vi "peak detector logic tester.vi"() -> ()   [LabVIEW 2021]
uses:
  <vilib>/rvi/FXPMathLib/FxpRectToPolar/subVIs/nifxpmath_RectToPolar_SimConfig.ctl
  <vilib>/rvi/Emulation/niFpgaSctlEmulationGetInTimedLoop.vi
  <vilib>/rvi/FXPMathLib/FxpRectToPolar/simVIs/DllFxpRectToPolarTemp_sub.vi
  <vilib>/rvi/Memory/Memory_Emulation/nirvimemoryFastEmulation.vi
  <vilib>/rvi/Memory/Memory_Emulation/nirvimemoryEmulation.vi
  <vilib>/rvi/Emulation/niFpgaEmulationIsFPGAContextNoSignature.vi
  <vilib>/rvi/DataTransferAndStorage/Container/Common/niFpgaContainerGetUniqueNameForEmu.vi
  <vilib>/rvi/Emulation/niFpgaProcessEmulError.vi
  <vilib>/rvi/errors/nirviReportUnexpectedCaseInternalError (U32).vi
  <vilib>/rvi/FXPMathLib/FxpRectToPolar/XNode/nifxpmath_RectToPolar.xnode
  <vilib>/rvi/DataTransferAndStorage/Container/XNode/niFpgaContainer.xnode
panel:
  out "addres 3":u32[](graph)
  out "addres 2":u16[](graph)
  out "amp":dbl[](graph)
  out "addres":u16[](graph)
  out "detected":dbl[](graph)
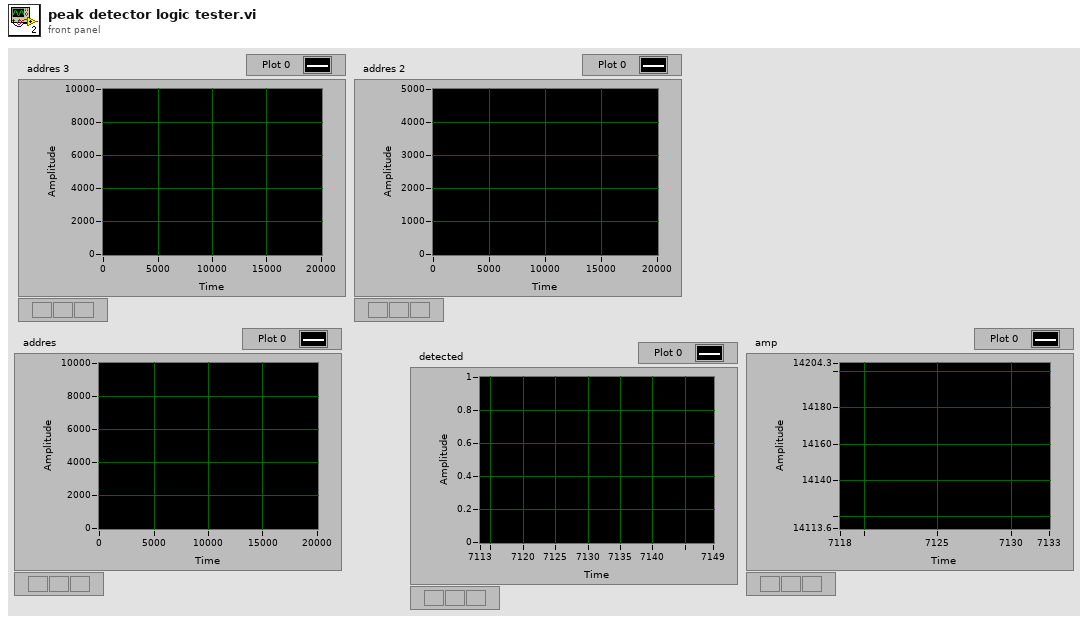
[diagram p1: front panel]
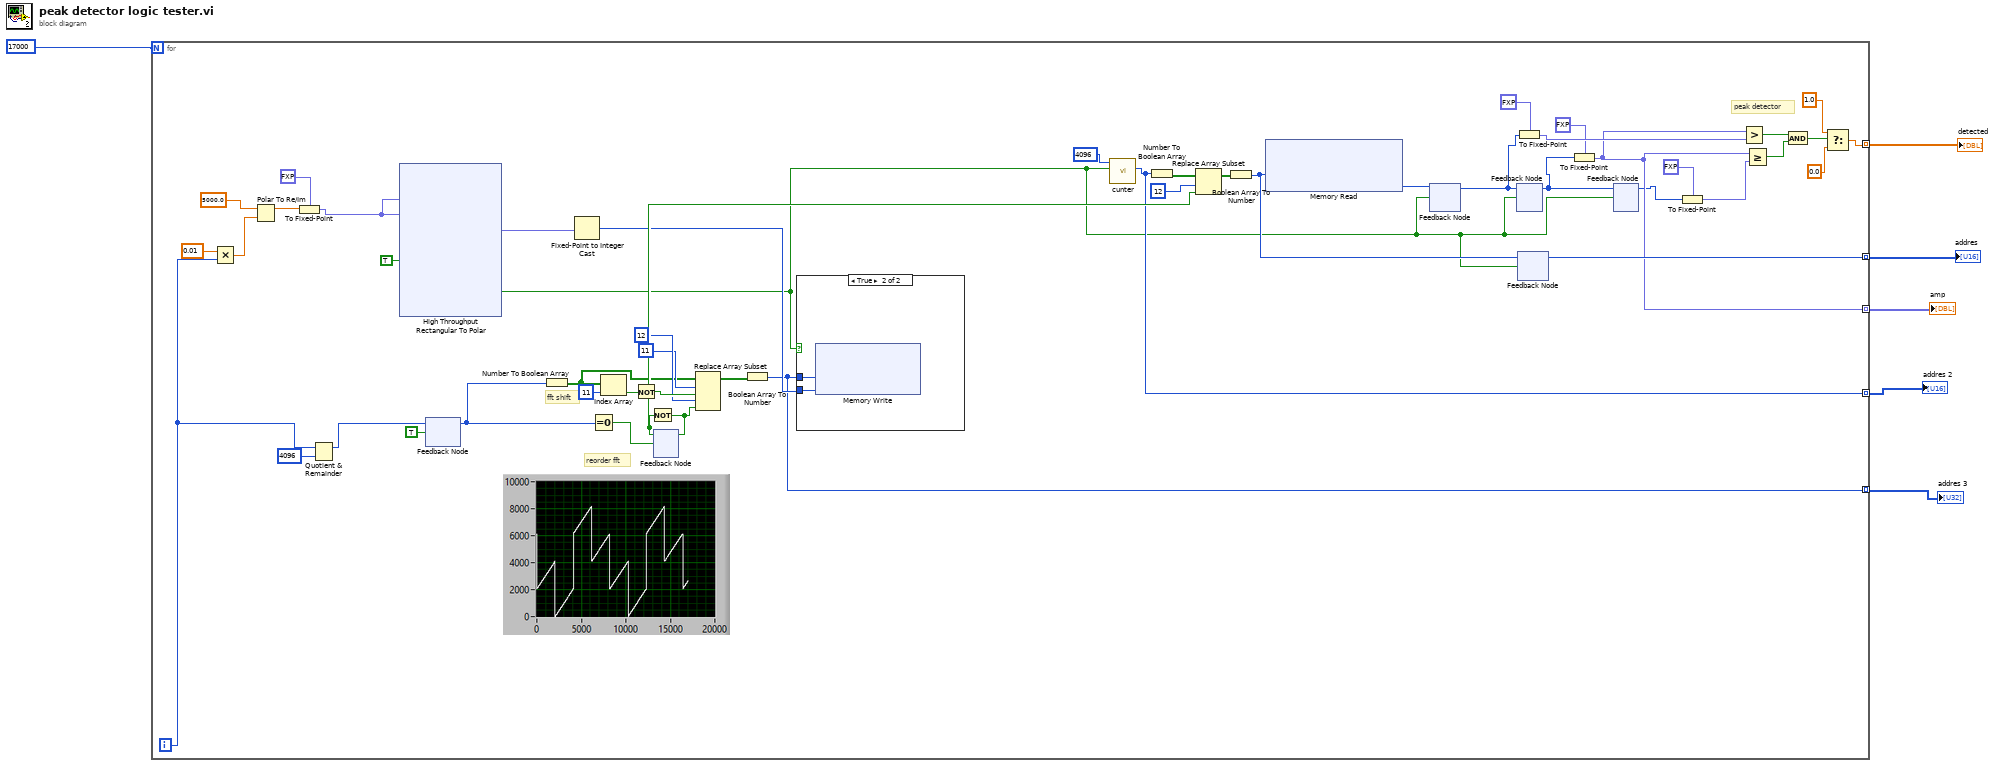
[diagram p0: block diagram]
diagram:
  n1 = for {
    N: 17000 -> [_]
    tunnel: [w29] -> w5 mode=indexing
    tunnel: [w26] -> w4 mode=indexing
    tunnel: [w15] -> w3 mode=indexing
    tunnel: [w10] -> w2 mode=indexing
    tunnel: [w9] -> w1 mode=indexing
    i -> [w25]
    # "reorder fft"
    # "peak detector"
    # "fft shift"
    n2 = Multiply(x=0.01, y=w25) -> (x*y=w35:dbl)
    n3 = Polar To Re/Im(2:w35, 3:5000.0 ("r")) -> (1:w33:dbl)  [unwired: 1 out]
    n4 = To Fixed-Point(fixed-point type=fxp<+/-,32,31> 0.0 ("x"), number=w33) -> (fixed-point=w31:fxp<+/-,32,31>)
    n5 = Quotient & Remainder(x=w25, y=4096) -> (x-y*floor(x/y)=w24:i32)  [unwired: 1 out]
    n6 = xnode "High Throughput Rectangular To Polar"("x"=w31, "y"=w31, "input valid"=TRUE) -> ("magnitude"=w47:fxp<+,32,31>, "output valid"=w7:bool)  [unwired: 1 in, 2 out]
    n7 = feedback #1() -> (w22:i32)  [unwired: 1 in]
    n8 = feedback-in #1(w24, TRUE) -> ()
    n9 = Number To Boolean Array(number=w22) -> (Boolean array=w39:bool[])
    n10 = Fixed-Point to Integer Cast(1:w47) -> (0:w48:u32)
    n11 = Equal To 0?(x=w22) -> (x = 0?=w43:bool)
    n12 = Index Array(array=w39, index=11) -> (element=w38:bool)
    n13 = Not(x=w38) -> (.not. x?=w44:bool)
    n14 = feedback #2() -> (w55:bool)  [unwired: 1 in]
    n15 = Not(x=w55) -> (.not. x?=w45:bool)
    n16 = feedback-in #2(w45, w43) -> ()
    n17 = Replace Array Subset(array=w39, new element #1=w44, index #1=11 ("index"), new element #2=w45, index #2=12 ("index")) -> (w46:bool[])
    n18 = Boolean Array To Number(Boolean array=w46) -> (number=w9:u32)
    n19 = case shown="True" w7 {
      tunnel: w9 -> [_ w57]
      tunnel: w48 -> [_ w56]
      frame False {
      }
      frame True {
        n20 = xnode "Memory Write"("Address"=w57, "Data"=w56) -> ()  [unwired: 1 in, 1 out]
      }
    }
    n21 = call "cunter.vi"("input valid"=w7, "count to"=u16 4096) -> ("count"=w10:u16)  [unwired: 8 in, 1 out]
    n22 = Number To Boolean Array(number=w10) -> (Boolean array=w50:bool[])
    n23 = Replace Array Subset(array=w50, new element=w55, index=12) -> (w51:bool[])
    n24 = Boolean Array To Number(Boolean array=w51) -> (number=w8:u16)
    n25 = xnode "Memory Read"("Address"=w8) -> ("Data"=w53:u32)  [unwired: 1 in, 1 out]
    n26 = feedback #3() -> (w18:u32)  [unwired: 1 in]
    n27 = feedback-in #3(w53, w7) -> ()
    n28 = To Fixed-Point(fixed-point type=fxp<+/-,32,31> 0.0 ("x"), number=w18) -> (fixed-point=w17:fxp<+/-,32,31>)
    n29 = feedback #4() -> (w14:u32)  [unwired: 1 in]
    n30 = feedback-in #4(w18, w7) -> ()
    n31 = feedback #5() -> (w26:u16)  [unwired: 1 in]
    n32 = feedback-in #5(w8, w7) -> ()
    n33 = To Fixed-Point(fixed-point type=fxp<+/-,32,31> 0.0 ("x"), number=w14) -> (fixed-point=w15:fxp<+/-,32,31>)
    n34 = feedback #6() -> (w12:u32)  [unwired: 1 in]
    n35 = feedback-in #6(w14, w7) -> ()
    n36 = To Fixed-Point(fixed-point type=fxp<+/-,32,31> 0.0 ("x"), number=w12) -> (fixed-point=w11:fxp<+/-,32,31>)
    n37 = Greater?(x=w15, y=w17) -> (0:w37:bool)
    n38 = Greater Or Equal?(x=w15, y=w11) -> (x >= y?=w54:bool)
    n39 = Compound Arithmetic op=AND(w37, w54) -> (w30:bool)
    n40 = Select(t=1.0, s=w30, f=0.0) -> (s? t:f=w29:dbl)
  }
  "detected" <- w5
  "addres" <- w4
  "amp" <- w3
  "addres 2" <- w2
  "addres 3" <- w1
